vi "Search By Name Path.vi"(10 "Node Name Path":string, 11 "Tree Map In":T1) -> (3 "Unique Paths Set":set{string}(c389))   [LabVIEW 2020, in "Tree Map.lvlib"]
doc: "Search the Tree Map for all unique node paths conforming with the special name path input. Each level of the special name path will be used for name search on that level of the tree.\n\nBecause this is a search operation, not a lookup operation, it is less efficient and should be used with caution. The performance will degrade with the size of the Tree Map.\n\n<b>Author:</b> Piotr Kruczkowski <PrimaryKey>\n<b>License:</b> NewBSD\n\nCopyright (c) 2019, National Instruments\nAll rights reserved.\n\nRedistribution and use in source and binary forms, with or without\nmodification, are permitted provided that the following conditions are met:\n1. Redistributions of source code must retain the above copyright\n notice, this list of conditions and the following disclaimer.\n2. Redistributions in binary form must reproduce the above copyright\n notice, this list of conditions and the following disclaimer in the\n documentation and/or other materials provided with the distribution.\n3. Neither the name of National Instruments nor the\n names of its contributors may be used to endorse or promote products\n derived from this software without specific prior written permission.\n\nTHIS SOFTWARE IS PROVIDED BY National Instruments ''AS IS'' AND ANY\nEXPRESS OR IMPLIED WARRANTIES, INCLUDING, BUT NOT LIMITED TO, THE IMPLIED\nWARRANTIES OF MERCHANTABILITY AND FITNESS FOR A PARTICULAR PURPOSE ARE\nDISCLAIMED. IN NO EVENT SHALL National Instruments BE LIABLE FOR ANY\nDIRECT, INDIRECT, INCIDENTAL, SPECIAL, EXEMPLARY, OR CONSEQUENTIAL DAMAGES\n(INCLUDING, BUT NOT LIMITED TO, PROCUREMENT OF SUBSTITUTE GOODS OR SERVICES;\nLOSS OF USE, DATA, OR PROFITS; OR BUSINESS INTERRUPTION) HOWEVER CAUSED AND\nON ANY THEORY OF LIABILITY, WHETHER IN CONTRACT, STRICT LIABILITY, OR TORT\n(INCLUDING NEGLIGENCE OR OTHERWISE) ARISING IN ANY WAY OUT OF THE USE OF THIS\nSOFTWARE, EVEN IF ADVISED OF THE POSSIBILITY OF SUCH DAMAGE."
uses:
  Tree Map.lvlib
  Tree Map Data.ctl
  b96954c2-77ba-4262-a89e-2345eefbb228.vi
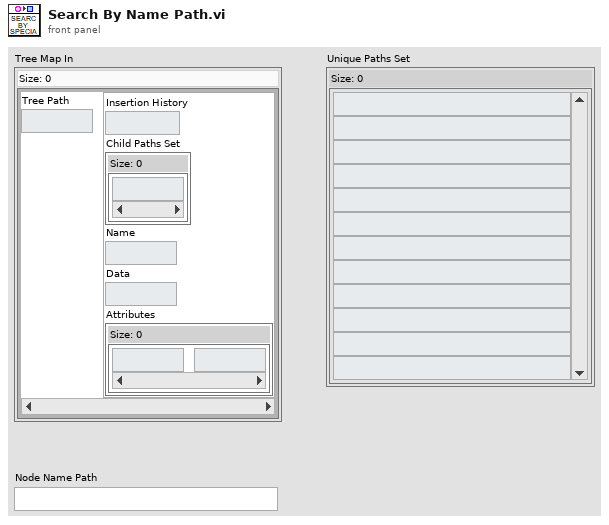
[diagram p1: front panel]
types:
  T1 = typedef "Tree Map.lvlib/Tree Map Data.ctl" = map{string, cluster{"Insertion History":i32, "Child Paths Set":set{string}, "Name":string, "Data":string, "Attributes":map{string, string}}}
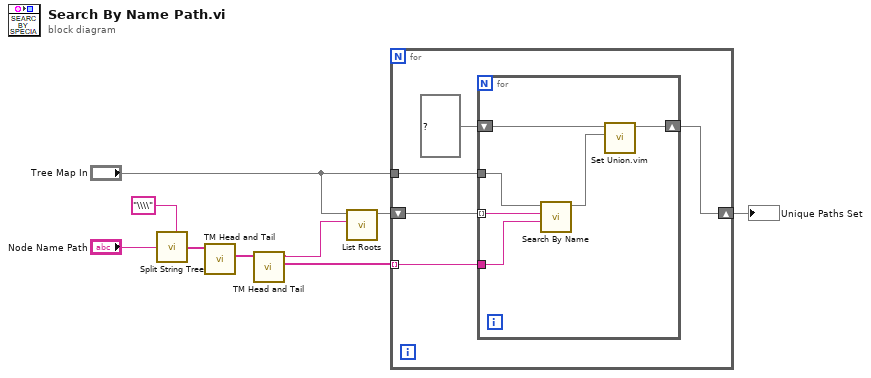
[diagram p0: block diagram]
diagram:
  n1 = call "Split String Tree.vi"("Split Pattern"="\\\\", "Input String"="Node Name Path") -> ("Split String"=w4:string[])  [unwired: 5 in]
  n2 = call "TM Head and Tail.vi"("List"=w4) -> ("Tail List"=w3:string[])  [unwired: 9 in, 1 out]
  n3 = call "TM Head and Tail.vi"("List"=w3) -> ("Tail List"=w1:string[], "Head"=w2:string)  [unwired: 9 in]
  n4 = call "List Roots.vi"("Optional Root Name"=w2, "Tree Map In"="Tree Map In") -> ("Unique Root Paths Set"=w6:set{string})  [unwired: 8 in, 1 out]
  n5 = for {
    tunnel: "Tree Map In" -> [w13]
    shift-right: [w10] -> w5
    shift-left: w6 -> [w14]
    tunnel: w1 -> [w12] mode=indexing
    n6 = for {
      tunnel: w14 -> [w20] mode=indexing
      tunnel: w13 -> [w19]
      shift-right: [w16] -> w10
      shift-left: set{string} {} ("union") -> [w18]
      tunnel: w12 -> [w15]
      n7 = call "Search By Name.vi"("Node Name"=w15, "Optional Unique Parent Path"=w20, "Tree Map In"=w19) -> ("Unique Paths Set"=w17:set{string})  [unwired: 8 in]
      n8 = call "Set Union.vim"("set 2"=w17, "set 1"=w18) -> ("union"=w16:set{string})  [unwired: 9 in]
    }
  }
  "Unique Paths Set" <- w5
